vi "final.vi"() -> ()   [LabVIEW 2016]
uses:
  <vilib>/Analysis/2dsp.llb/1D Convolution (DBL).vi
  <vilib>/Analysis/NI_AALBase.lvlib
  <vilib>/Analysis/NI_AALPro.lvlib
  usr/local/lib/libcirc.so
panel:
  out "Input":dbl[](graph)
  in  "f2 for Chirp":dbl=0.5 format="%0.2f"
  in  "frequency":dbl=0.0078125 format="%0.4e"
  in  "amplitude":dbl=1.0 format="%0.2f"
  in  "Case":dbl
  in  "milliseconds to wait":u32
  in  "stop":bool
  out "LinearToTest":dbl[](graph)
  out "OverLapAndSav":sgl[](graph)
  out "fin_img 2":sgl[](array[numeric])
  out "fin_real 2":sgl[](array[numeric])
  in  "flt_size":i32
  in  "inp_size":i32
  in  "h_real":sgl[](array[numeric])
  in  "L":i32
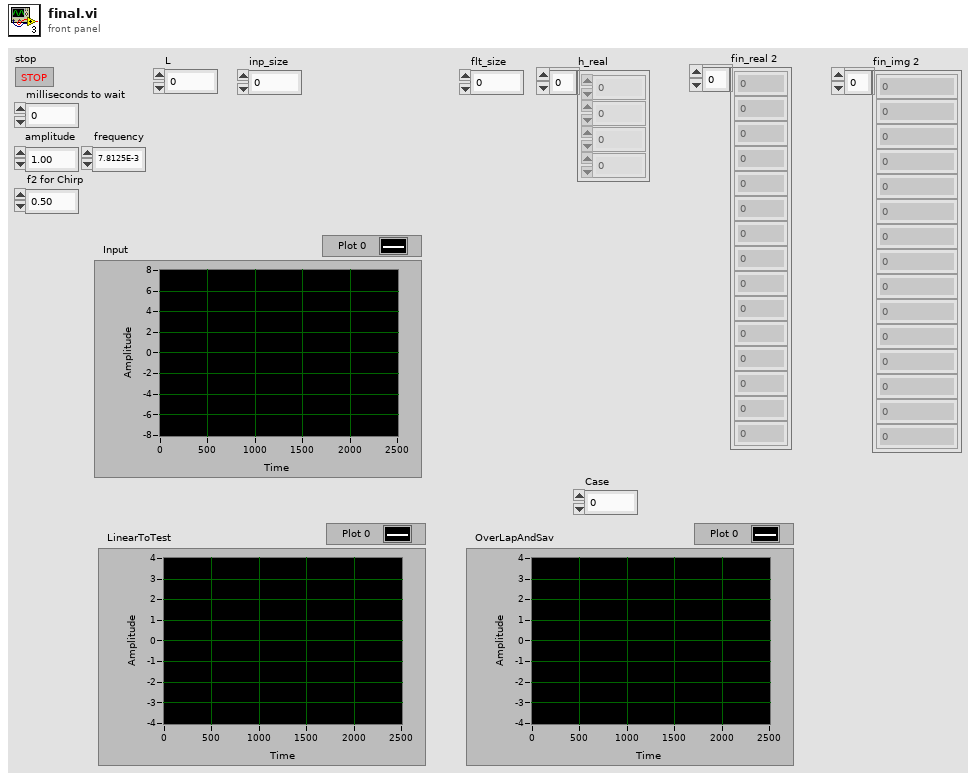
[diagram p1: front panel]
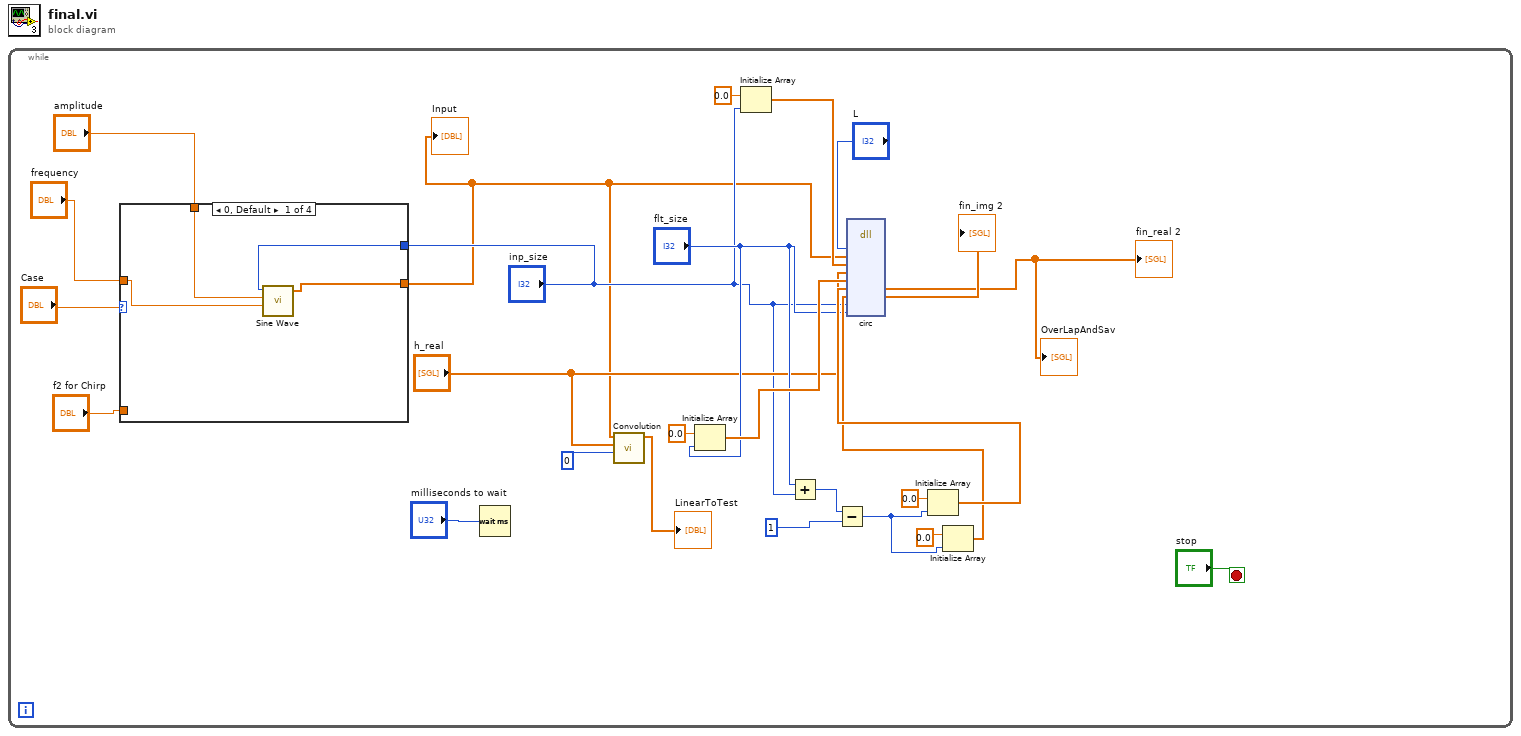
[diagram p0: block diagram]
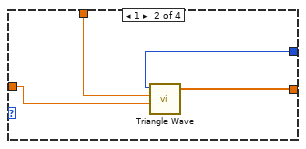
[diagram p2: hidden frame]
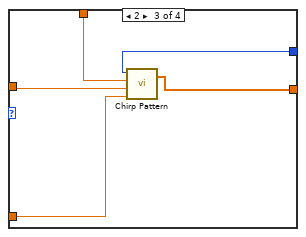
[diagram p3: hidden frame]
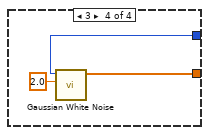
[diagram p4: hidden frame]
diagram:
  n1 = while {
    stop <- "stop" stop-if-true
    n2 = case shown="0, Default" "Case" {
      tunnel: [w30 w33 w39 w41] -> w1
      tunnel: "inp_size" -> [w29 w34 w38 w40]
      tunnel: "amplitude" -> [w28 w32 w37 _]
      tunnel: "frequency" -> [w27 w31 w36 _]
      tunnel: "f2 for Chirp" -> [_ _ w35 _]
      frame 0, Default {
        n3 = call <vilib>:"Sine Wave.vi"("samples"=w29, "amplitude"=w28, "frequency"=w27) -> ("sine wave"=w30:dbl[])  [unwired: 2 in, 2 out]
      }
      frame 1 {
        n4 = call <vilib>:"Triangle Wave.vi"("samples"=w34, "amplitude"=w32, "frequency"=w31) -> ("triangle wave"=w33:dbl[])  [unwired: 2 in, 2 out]
      }
      frame 2 {
        n5 = call <vilib>:"Chirp Pattern.vi"("f2"=w35, "f1"=w36, "amplitude"=w37, "samples"=w38) -> ("Chirp Pattern"=w39:dbl[])  [unwired: 1 out]
      }
      frame 3 {
        n6 = call <vilib>:"Gaussian White Noise.vi"("standard deviation"=2.0, "samples"=w40) -> ("Gaussian noise pattern"=w41:dbl[])  [unwired: 8 in, 1 out]
      }
    }
    "Input" <- w1
    n7 = Wait (ms)(milliseconds to wait="milliseconds to wait") -> ()  [unwired: 1 out]
    n8 = call-poly <vilib>:"Convolution.vi"("algorithm"=0 ("y"), "Y"="h_real", "X"=w1) -> ("X * Y"=→"LinearToTest":dbl[])  [unwired: 7 in, 1 out]
    n9 = Initialize Array(0.0 ("element"), "flt_size") -> (w14:dbl[])
    n10 = Initialize Array(0.0 ("element"), "inp_size") -> (w16:dbl[])
    n11 = Add(x="flt_size", y="inp_size") -> (x+y=w22:i32)
    n12 = Subtract(x=w22, y=1) -> (x-y=w20:i32)
    n13 = Initialize Array(0.0 ("element"), w20) -> (w19:dbl[])
    n14 = Initialize Array(0.0 ("element"), w20) -> (w18:dbl[])
    n15 = dll-call lib="usr/local/lib/libcirc.so" fn="circ"("L"="L", "input_real"=w1, "input_img"=w16, "h_real"="h_real", "h_img"=w14, "fin_real"=w19, "fin_img"=w18, "inp_size"="inp_size", "flt_size"="flt_size") -> ("fin_real"=→"fin_real 2" →"OverLapAndSav":sgl[], "fin_img"=→"fin_img 2":sgl[])  [unwired: 11 in, 2 out]
  }
